vi "5 ch 8or12kHz resonance scanner (FPGA) fixed pix clock.vi"() -> ()   [LabVIEW 2012]
uses:
  <vilib>/Platform/TimedLoop/XDataNode/timing_clust.ctl
  <vilib>/Platform/TimedLoop/XDataNode/nitl_modes.ctl
  <vilib>/Platform/TimedLoop/XDataNode/wakeup.ctl
  <vilib>/rvi/eio/common/nirviEmuTemplateMethod_errors.vi
  <vilib>/rvi/Emulation/niFpgaSctlEmulationRegisterWithScheduler.vi
  <vilib>/rvi/interface/RandomDataEmulation/nirviRandomDataFPGAFIFO.vi
  <vilib>/rvi/interface/RandomDataEmulation/niFpgaRandomDataHandleErrors.vi
  <vilib>/rvi/Emulation/niFpgaSctlEmulationScheduler.vi
  <vilib>/eio/EIONode/EIONode.xnode
  <vilib>/platform/TimedLoop/XDataNode/XDataNode.xnode
  <vilib>/rvi/DataTransferAndStorage/Container/XNode/niFpgaContainer.xnode
  <vilib>/rvi/interface/RandomDataEmulation/nirviRandomDataFpgaReadWriteTemplate.vi
  <vilib>/Platform/TimedLoop/XDataNode/XDNodeRunTimeDep.lvlib
panel:
  in  "frequency (T:8kHz F:12kHz)":bool
  in  "lines at once":i16=4999
  in  "Start Delay (Ticks)":i16 caption="Start delay (Ticks)"
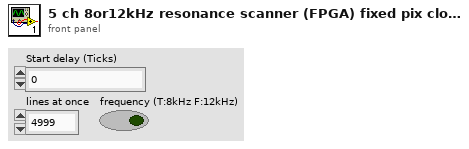
[diagram p1: front panel]
types:
  T1 = typedef "XDNodeRunTimeDep.lvlib/timing_clust.ctl" = cluster{"Expected End [f-1]":u64, "Actual End [f-1]":u64, "Finished Late? [f-1]":bool, "Expected End [i-1]":u64, "Actual End [i-1]":u64, "Finished Late? [i-1]":bool, "Expected Start [i]":u64, "Actual Start [i]":u64, "Expected Start [f]":u64, "Actual Start [f]":u64, "Source Name":string, "Structure Name":string, "Period":i64, "Deadline":i64, "Offset":i64, "Start":i64, "Priority":i32, "Timeout":i32, "Mode":T2, "Wakeup Reason":T3, "Error":errorcluster, "Source Type":string, "Secondary Source Type":string, "Global End Time":u64, "Global Start Time":u64, "Frame Duration":u64, "Iteration Duration":u64, "Assigned CPU":i32, "I/O Scan Engine Mode":u32}
  T2 = typedef "XDNodeRunTimeDep.lvlib/nitl_modes.ctl" = enum32{"No Change", "Process missed periods, maintain original phase", "Discard missed periods, maintain original phase", "Process missed periods, ignore original phase", "Discard missed periods, ignore original phase"}
  T3 = typedef "XDNodeRunTimeDep.lvlib/wakeup.ctl" = enum32{"Normal", "Aborted", "Asynchronous wakeup", "Timing source error", "Timed loop error", "Timeout"}
  T4 = cluster{"IO Module\\AI A0":i32, "IO Module\\AI A1":i32, "IO Module\\AI A3":i32, "IO Module\\AI A6":i32, "IO Module\\AI B8":i32}
  T5 = cluster{"IO Module\\AI A0":i16, "IO Module\\AI A1":i16, "IO Module\\AI A3":i16, "IO Module\\AI A6":i16, "IO Module\\AI B8":i16}
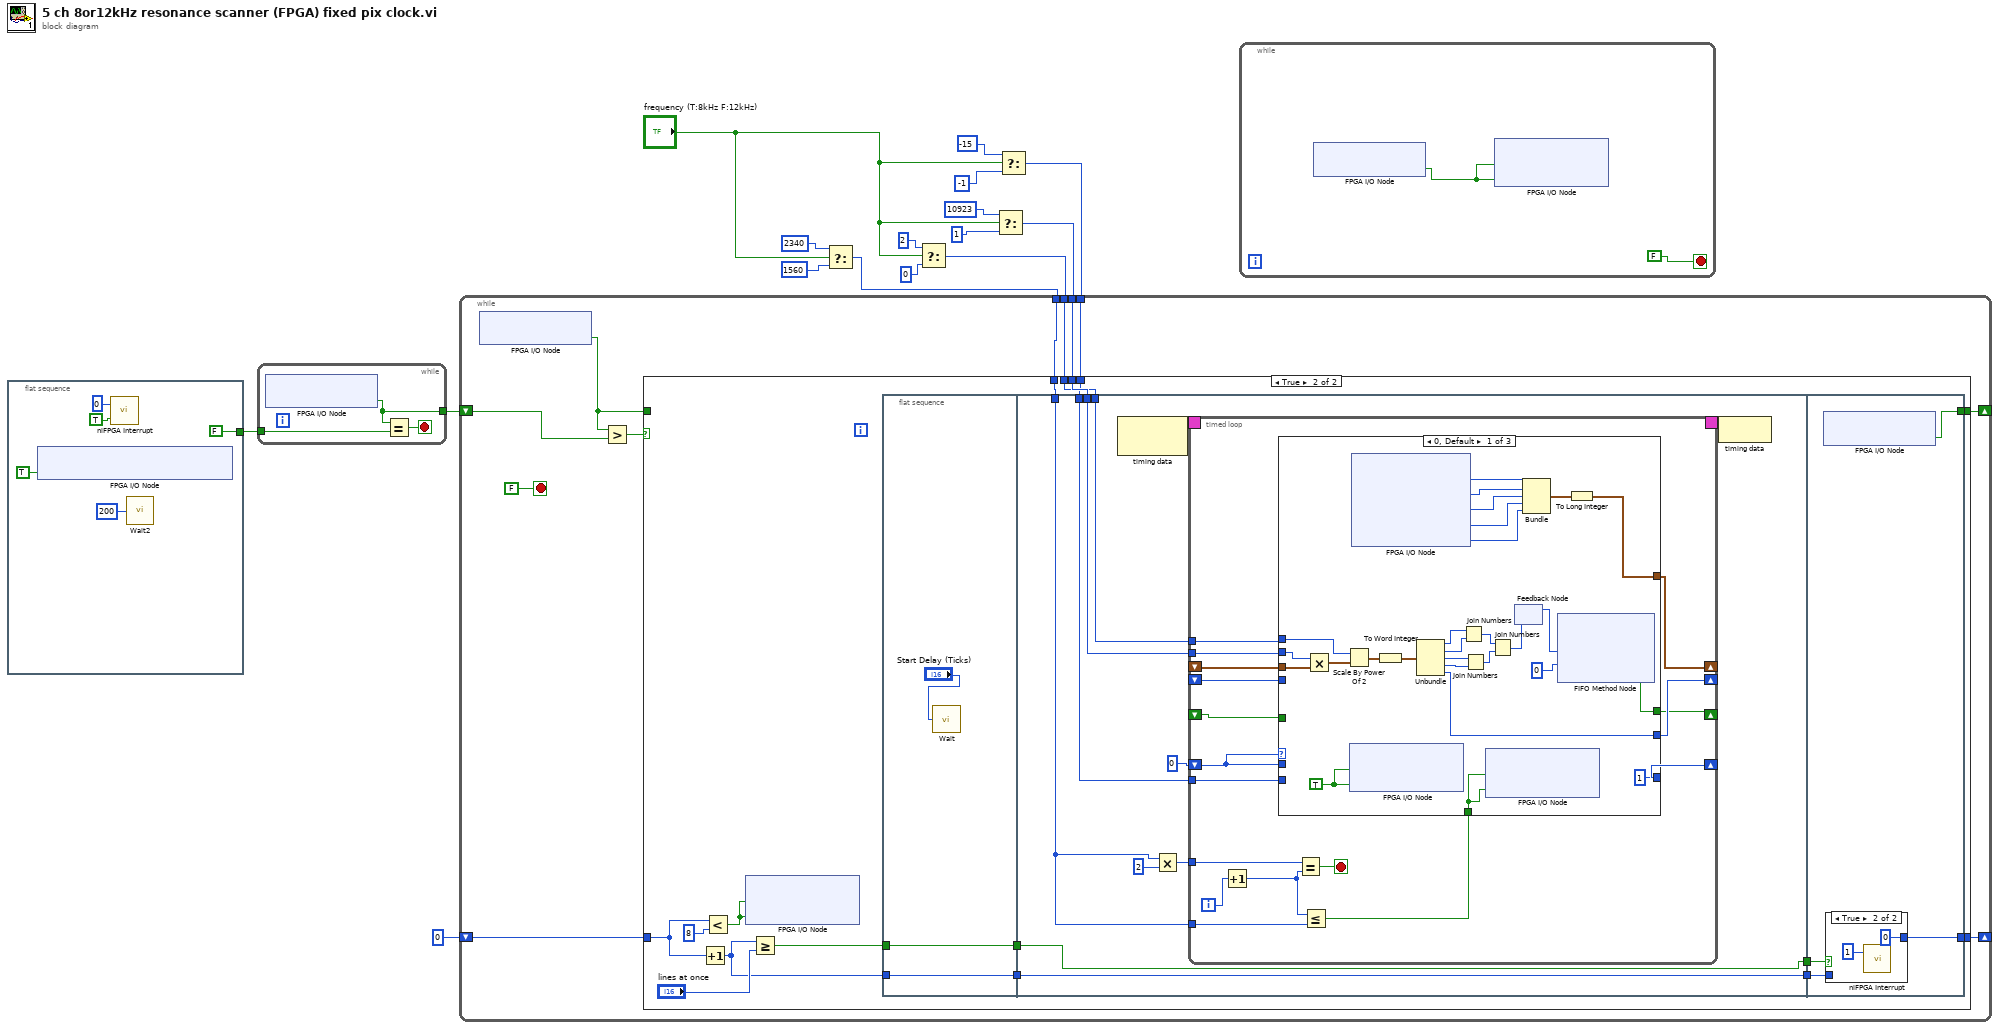
[diagram p0: block diagram]
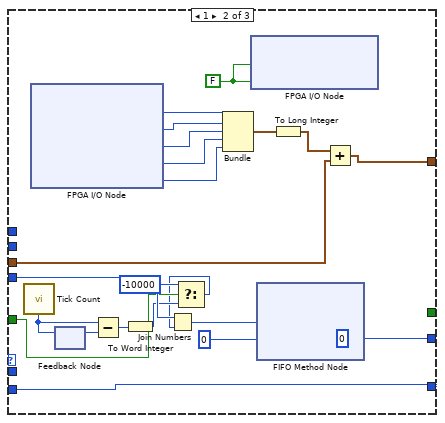
[diagram p3: hidden frame]
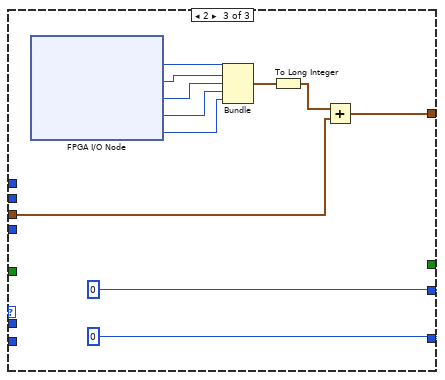
[diagram p4: hidden frame]
diagram:
  n1 = flat-sequence {
    tunnel: [FALSE ("IO Module\\DI 0")] -> w15
    frame #0 {
      n2 = xnode "FPGA I/O Node"("IO Module\\Digital Output Enable"=TRUE ("IO Module\\Digital Output Enable")) -> ()  [unwired: 1 in, 1 out]
      n3 = call <vilib>:"niFPGA Interrupt.vi"("Wait Until Cleared (F)"=TRUE, "IRQ Number (0)"=u8 0) -> ()  [unwired: 1 in]
      n4 = call "Wait2"("Count(mSec)"=u32 200) -> ()  [unwired: 1 out]
    }
  }
  n5 = while {
    tunnel: w15 -> [w24]
    tunnel: [w22] -> w14
    stop <- w23 stop-if-true
    n6 = xnode "FPGA I/O Node"() -> ("IO Module\\DI 0"=w22:bool)  [unwired: 1 in, 1 out]
    n7 = Equal?(x=w22, y=w24) -> (x = y?=w23:bool)
  }
  n8 = Select(t=i16 2340 ("samples per half period"), s="frequency (T:8kHz F:12kHz)", f=i16 1560 ("samples per half period")) -> (s? t:f=w1:i16)
  n9 = Select(t=i8 2 ("f"), s="frequency (T:8kHz F:12kHz)", f=i8 0 ("n")) -> (s? t:f=w5:i8)
  n10 = Select(t=i16 10923 ("n"), s="frequency (T:8kHz F:12kHz)", f=i16 1) -> (s? t:f=w7:i16)
  n11 = Select(t=i16 -15 ("n"), s="frequency (T:8kHz F:12kHz)", f=i16 -1 ("n")) -> (s? t:f=w6:i16)
  n12 = while {
    shift-right: [w34] -> _
    shift-left: w14 -> [w35]
    shift-right: [w32] -> _
    shift-left: i16 0 ("IRQ Number (0)") -> [w31]
    tunnel: w7 -> [w29]
    tunnel: w6 -> [w28]
    tunnel: w5 -> [w27]
    tunnel: w1 -> [w26]
    stop <- FALSE stop-if-true
    n13 = xnode "FPGA I/O Node"() -> ("IO Module\\DI 0"=w25:bool)  [unwired: 1 in, 1 out]
    n14 = Greater?(x=w25, y=w35) -> (0:w30:bool)
    n15 = case shown="True" w30 {
      tunnel: [w36 w50] -> w34
      tunnel: w31 -> [w37 w52]
      tunnel: [w37 w53] -> w32
      tunnel: w25 -> [w36 _]
      tunnel: w29 -> [_ w49]
      tunnel: w28 -> [_ w48]
      tunnel: w27 -> [_ w47]
      tunnel: w26 -> [_ w46]
      frame False {
      }
      frame True {
        n16 = Increment(x=w52) -> (x+1=w41:i16)
        n17 = Less?(x=w52, y=i16 8) -> (x < y?=w45:bool)
        n18 = xnode "FPGA I/O Node"("PXI_Trig2"=w45, "IO Module\\D0 2"=w45) -> ()  [unwired: 2 in, 2 out]
        n19 = Greater Or Equal?(x=w41, y="lines at once") -> (x >= y?=w38:bool)
        n20 = flat-sequence {
          tunnel: [w55] -> w42
          tunnel: w41 -> [w55]
          tunnel: [w54] -> w39
          tunnel: w38 -> [w54]
          tunnel: w49 -> [w62]
          tunnel: w48 -> [w61]
          tunnel: w47 -> [w60]
          tunnel: w46 -> [w59]
          tunnel: [w58] -> w43
          tunnel: w42 -> [w58]
          tunnel: [w57] -> w40
          tunnel: w39 -> [w57]
          tunnel: [w152] -> w53
          tunnel: [w151] -> w50
          tunnel: w43 -> [w150]
          tunnel: w40 -> [w149]
          frame #0 {
            n21 = call "Wait"("Count(Ticks)"="Start Delay (Ticks)") -> ()  [unwired: 1 out]
          }
          frame #1 {
            n22 = node-c288() -> (w65:T1)  [unwired: 1 in]
            n23 = Multiply(x=w59, y=i16 2) -> (x*y=w66:i16)
            n24 = timed-loop {
              tunnel: w66 -> [w83]
              timing: w65 -> [_]
              timing-out: [_] -> w64
              shift-right: [w82] -> _
              shift-left: i8 0 ("Timeout") -> [w74]
              tunnel: w59 -> [w80]
              shift-right: [w78] -> _
              shift-left: _ -> [w77]
              shift-right: [w76] -> _
              shift-left: _ -> [w75]
              tunnel: w62 -> [w73]
              tunnel: w61 -> [w72]
              tunnel: w60 -> [w71]
              shift-right: [w70] -> _
              shift-left: _ -> [w69]
              i -> [w79]
              stop <- w84 stop-if-true
              n25 = Increment(x=w79) -> (x+1=w81:i32)
              n26 = Equal?(x=w83, y=w81) -> (x = y?=w84:bool)
              n27 = Less Or Equal?(x=w81, y=w80) -> (x <= y?=w68:bool)
              n28 = case shown="0, Default" w74 {
                tunnel: w74 -> [_ _ _]
                tunnel: [i8 1 w113 i8 0] -> w82
                tunnel: [w105 w125 w136] -> w78
                tunnel: w77 -> [w95 w126 w137]
                tunnel: [w92 i16 0 ("IO Module\\AI B8") i16 0 ("IO Module\\AI B8")] -> w76
                tunnel: w75 -> [_ w120 _]
                tunnel: w73 -> [w94 _ _]
                tunnel: w72 -> [w93 _ _]
                tunnel: w71 -> [_ w113 _]
                tunnel: [w90 _ _] -> w70
                tunnel: w69 -> [_ w116 _]
                tunnel: w68 -> [w85 _ _]
                frame 0, Default {
                  w86 = TRUE ("PXI_Trig1")
                  n29 = Multiply(x=w94, y=w95) -> (x*y=w97:T4)
                  n30 = Scale By Power Of 2(n=w93, x=w97) -> (x*2^n=w96:T4)
                  n31 = xnode "FPGA I/O Node"("IO Module\\D0 0"=w86, "PXI_Trig0"=w86) -> ()  [unwired: 2 in, 2 out]
                  n32 = xnode "FPGA I/O Node"() -> ("IO Module\\AI A0"=w111:i16, "IO Module\\AI A1"=w110:i16, "IO Module\\AI A3"=w109:i16, "IO Module\\AI A6"=w108:i16, "IO Module\\AI B8"=w106:i16)  [unwired: 5 in, 5 out]
                  n33 = To Word Integer(number=w96) -> (16bit integer=w87:T5)
                  n34 = Unbundle(w87) -> ("IO Module\\AI A0"=w101:i16, "IO Module\\AI A1"=w100:i16, "IO Module\\AI A3"=w99:i16, "IO Module\\AI A6"=w98:i16, "IO Module\\AI B8"=w92:i16)
                  n35 = Join Numbers(hi=w101, lo=w100) -> ((hi.lo)=w102:u32)
                  n36 = Join Numbers(hi=w99, lo=w98) -> ((hi.lo)=w103:u32)
                  n37 = xnode "FPGA I/O Node"("IO Module\\D0 1"=w85, "PXI_Trig1"=w85) -> ()  [unwired: 2 in, 2 out]
                  n38 = Join Numbers(hi=w102, lo=w103) -> ((hi.lo)=w91:u64)
                  n39 = feedback-in #1(w91) -> ()
                  n40 = feedback #1() -> (w89:u64)  [unwired: 1 in]
                  n41 = Bundle("IO Module\\AI A0"=w111, "IO Module\\AI A1"=w110, "IO Module\\AI A3"=w109, "IO Module\\AI A6"=w108, "IO Module\\AI B8"=w106) -> (w107:T5)  [unwired: 1 in]
                  n42 = xnode ("FIFO Method Node")("Element"=w89, "Timeout"=0) -> ("Timed Out?"=w90:bool)  [unwired: 1 in, 1 out]
                  n43 = To Long Integer(number=w107) -> (32bit integer=w105:T4)
                }
                frame 1 {
                  w112 = FALSE ("PXI_Trig1")
                  n44 = call "Tick Count"() -> ("Tick Count(Ticks)"=w124:u32)
                  n45 = xnode "FPGA I/O Node"() -> ("IO Module\\AI A0"=w133:i16, "IO Module\\AI A1"=w132:i16, "IO Module\\AI A3"=w131:i16, "IO Module\\AI A6"=w130:i16, "IO Module\\AI B8"=w128:i16)  [unwired: 5 in, 5 out]
                  n46 = feedback #2() -> (w123:u32)  [unwired: 1 in]
                  n47 = feedback-in #2(w124) -> ()
                  n48 = Subtract(x=w124, y=w123) -> (x-y=w122:u32)
                  n49 = To Word Integer(number=w122) -> (16bit integer=w117:i16)
                  n50 = Select(t=i16 -10000, s=w116, f=w117) -> (s? t:f=w114:i16)
                  n51 = Join Numbers(hi=w120, lo=w114) -> ((hi.lo)=w118:u32)
                  n52 = Bundle("IO Module\\AI A0"=w133, "IO Module\\AI A1"=w132, "IO Module\\AI A3"=w131, "IO Module\\AI A6"=w130, "IO Module\\AI B8"=w128) -> (w129:T5)  [unwired: 1 in]
                  n53 = xnode "FPGA I/O Node"("IO Module\\D0 0"=w112, "PXI_Trig0"=w112) -> ()  [unwired: 2 in, 2 out]
                  n54 = xnode ("FIFO Method Node")("Element"=w118, "Timeout"=0) -> ()  [unwired: 1 in, 2 out]
                  n55 = To Long Integer(number=w129) -> (32bit integer=w127:T4)
                  n56 = Add(x=w127, y=w126) -> (x+y=w125:T4)
                }
                frame 2 {
                  n57 = xnode "FPGA I/O Node"() -> ("IO Module\\AI A0"=w144:i16, "IO Module\\AI A1"=w143:i16, "IO Module\\AI A3"=w142:i16, "IO Module\\AI A6"=w141:i16, "IO Module\\AI B8"=w139:i16)  [unwired: 5 in, 5 out]
                  n58 = Bundle("IO Module\\AI A0"=w144, "IO Module\\AI A1"=w143, "IO Module\\AI A3"=w142, "IO Module\\AI A6"=w141, "IO Module\\AI B8"=w139) -> (w140:T5)  [unwired: 1 in]
                  n59 = To Long Integer(number=w140) -> (32bit integer=w138:T4)
                  n60 = Add(x=w138, y=w137) -> (x+y=w136:T4)
                }
              }
            }
            n61 = node-c288(w64) -> ()
          }
          frame #2 {
            n62 = xnode "FPGA I/O Node"() -> ("IO Module\\DI 0"=w151:bool)  [unwired: 1 in, 1 out]
            n63 = case shown="True" w149 {
              tunnel: w150 -> [w153 _]
              tunnel: [w153 u8 0] -> w152
              frame False {
              }
              frame True {
                n64 = call <vilib>:"niFPGA Interrupt.vi"("IRQ Number (0)"=u8 1) -> ()  [unwired: 2 in]
              }
            }
          }
        }
      }
    }
  }
  n65 = while {
    stop <- FALSE stop-if-true
    n66 = xnode "FPGA I/O Node"() -> ("IO Module\\DI 0"=w157:bool)  [unwired: 1 in, 1 out]
    n67 = xnode "FPGA I/O Node"("IO Module\\D0 3"=w157, "PXI_Trig3"=w157) -> ()  [unwired: 2 in, 2 out]
  }
